vi "Configure Relative Measurement.vi"(7 "Enable Set Reference Value (F: Disable)":bool, 8 "error in (no error)":errorcluster, 9 "Measurement Number (1: Measurement 1)":i32(ring)=1 items=["Measurement 1"=1, "Measurement 2"=2, "Measurement 3"=3, "Measurement 4"=4], 10 "Enable Relaive Mode (F: Disable)":bool, 11 "VISA resource name":refnum<visa-resource-name>) -> (0 "error out":errorcluster, 3 "VISA resource name out":refnum<visa-resource-name>)   [LabVIEW 2011, in "Agilent N432A.lvlib"]
doc: "Compares the measurement signal to a reference value. The relative value is applied to the measurement signal after any math calculations and display offsets have been applied."
uses:
  <instrlib>/Agilent N432A/Agilent N432A.lvlib
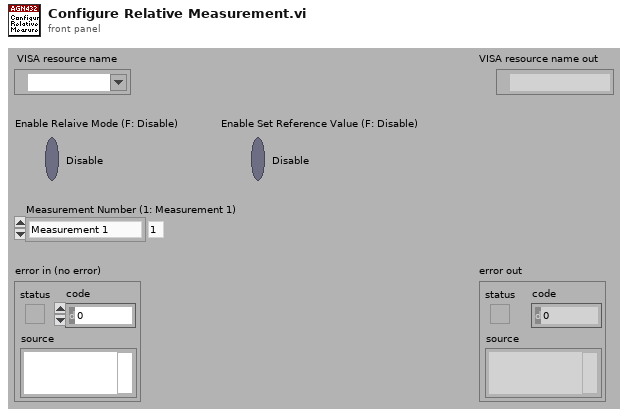
[diagram p1: front panel]
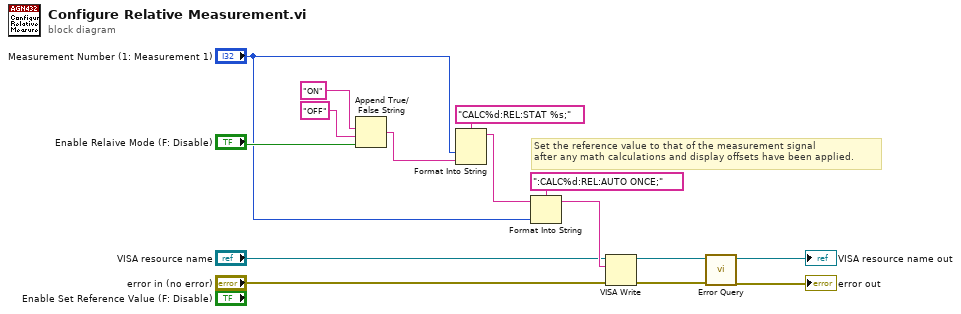
[diagram p0: block diagram]
diagram:
  # "Set the reference value to that of the measurement signal\nafter any math calculations and display offsets have been applied."
  n1 = Append True/False String(1:"Enable Relaive Mode (F: Disable)", 2:"OFF", 3:"ON") -> (0:w10:string)  [unwired: 1 in]
  n2 = Format Into String(format string="CALC%d:REL:STAT %s;", "Measurement Number (1: Measurement 1)", w10) -> (resulting string=w8:string)  [unwired: 2 in, 1 out]
  n3 = Format Into String(format string=":CALC%d:REL:AUTO ONCE;", initial string=w8, "Measurement Number (1: Measurement 1)") -> (resulting string=w7:string)  [unwired: 1 in, 1 out]
  n4 = VISA Write(VISA resource name="VISA resource name", write buffer=w7, error in (no error)="error in (no error)") -> (VISA resource name out=w4:refnum<visa-resource-name>, error out=w3:errorcluster)  [unwired: 1 out]
  n5 = call <instrlib>:"Error Query.vi"("error in (no error)"=w3, "VISA resource name"=w4) -> ("error out"=→"error out":errorcluster, "VISA resource name out"=→"VISA resource name out":refnum<visa-resource-name>)  [unwired: 6 in, 2 out]
